vi "createProcessSetting.vi"(8 "error in (no error)":errorcluster, 11 "Boot in":refnum<class "Boot.lvclass">) -> (0 "error out":errorcluster, 2 "ProcessSetting":refnum<class "Setting.lvclass">, 3 "Boot out":refnum<class "Boot.lvclass">)   [LabVIEW 2016, in "Boot.lvclass"]
uses:
  Boot.lvclass
  Settings/Settings/Setting.lvclass
  Settings/ProcessSetting/ProcessSetting.lvclass
  D:/Code/ts_M1M3Support/Settings/Settings/Setting.lvclass
  Settings/Settings/Setting.lvclass/Setting.ctl
  Boot.lvclass/Boot.ctl
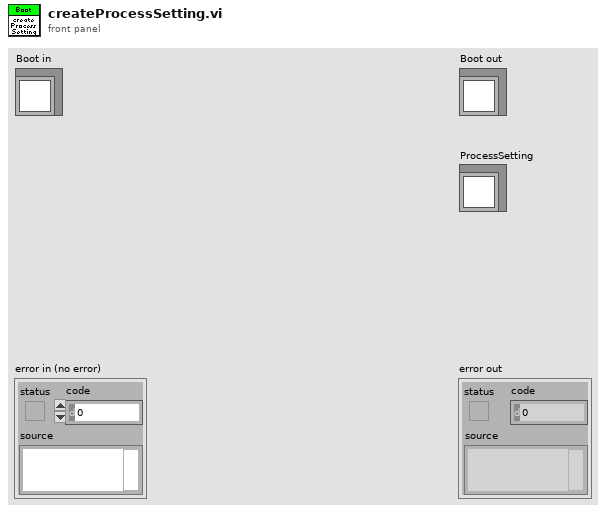
[diagram p1: front panel]
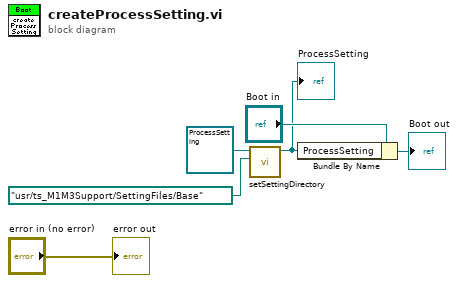
[diagram p0: block diagram]
diagram:
  n1 = call "setSettingDirectory.vi"("SettingDirectory"=path "/usr/ts_M1M3Support/SettingFiles/Base", "BaseSetting in"=refnum<class "ProcessSetting.lvclass"> refnum ("ProcessSetting.lvclass")) -> ("BaseSetting out"=w1:refnum<class "ProcessSetting.lvclass">)  [unwired: 9 in]
  "ProcessSetting" <- w1
  n2 = Bundle By Name(cluster="Boot in", "ProcessSetting"=w1) -> (→"Boot out":refnum<class "Boot.lvclass">)
  "error out" <- "error in (no error)"
